vi "subReadVersionFile.vi"(8 "error in":errorcluster) -> (0 "error out":errorcluster, 1 "Step Types Version":string, 2 "TestStand Versions":string)   [LabVIEW 2015, in "veristand-steps-build-tools.lvlib"]
uses:
  veristand-steps-build-tools.lvlib
  <vilib>/Utility/config.llb/Read Key (String).vi
  <vilib>/Utility/config.llb/NI_LVConfig.lvlib
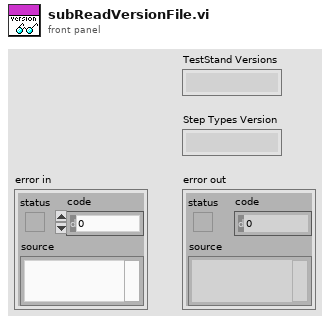
[diagram p1: front panel]
types:
  T1 = typedef "NI_LVConfig.lvlib/Config Data RefNum.ctl" = refnum<k1>
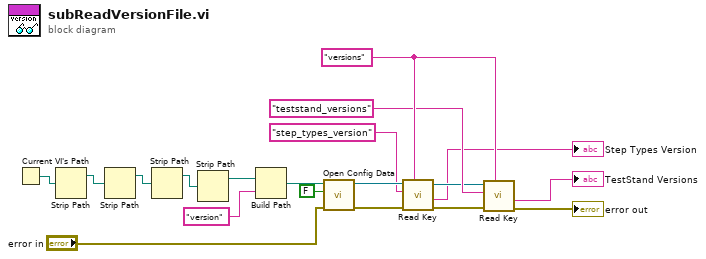
[diagram p0: block diagram]
diagram:
  w7 = "versions" ("section")
  n1 = Current VI's Path() -> (path=w19:path)
  n2 = Strip Path(path=w19) -> (stripped path=w18:path)  [unwired: 1 out]
  n3 = Strip Path(path=w18) -> (stripped path=w17:path)  [unwired: 1 out]
  n4 = Strip Path(path=w17) -> (stripped path=w15:path)  [unwired: 1 out]
  n5 = Strip Path(path=w15) -> (stripped path=w14:path)  [unwired: 1 out]
  n6 = Build Path(base path=w14, name or relative path="version") -> (appended path=w13:path)
  n7 = call <vilib>:"Open Config Data.vi"("error in (no error)"="error in", "create file if necessary (T)"=FALSE, "configuration file path"=w13) -> ("error out"=w10:errorcluster, "refnum"=w11:T1)  [unwired: 6 in, 1 out]
  n8 = call-poly <vilib>:"Read Key.vi"("section"=w7, "error in (no error)"=w10, "key"="step_types_version", "refnum"=w11) -> ("error out"=w8:errorcluster, "value"=→"Step Types Version":string, "refnum out"=w5:T1)  [unwired: 4 in, 1 out]
  n9 = call-poly <vilib>:"Read Key.vi"("section"=w7, "error in (no error)"=w8, "key"="teststand_versions", "refnum"=w5) -> ("error out"=→"error out":errorcluster, "value"=→"TestStand Versions":string)  [unwired: 4 in, 2 out]
